vi "Init Commands.vi"(8 "error in (no error)":errorcluster, 10 "Commands":refnum<class "Group Config.lvclass">, 11 "DAQmxAI in":refnum<class "DAQmxAI.lvclass">) -> (0 "error out":errorcluster, 3 "DAQmxAI out":refnum<class "DAQmxAI.lvclass">)   [LabVIEW 2023, in "VolatusDAQ.lvlib" / "DAQmxAI.lvclass"]
uses:
  DAQmxAI.lvclass
  C:/dev/volatus/mts-volatus-super/libs/lv-volatus/Volatus/Module/Module.lvclass
  VolatusConfig/Group/Group Config.lvclass
  lv-vecto/Vecto/Group DBL/Group DBL.lvclass
  C:/dev/volatus/mts-volatus-super/libs/lv-vecto/Vecto/Group/Group.lvclass
  Cmd Index.ctl
  VolatusConfig/VolatusConfigElement/VolatusConfigElement.lvclass/VolatusConfigElement.ctl
  DAQmxAI.lvclass/DAQmxAI.ctl
  VolatusConfig/VolatusConfigElement/Element.vi
  VolatusConfig/Channel/Channel Config.lvclass
  C:/dev/volatus/mts-volatus-super/libs/lv-volatus/VolatusConfig/VolatusConfigElement/VolatusConfigElement.lvclass
  VolatusConfig/VolatusConfigElement/VolatusConfigElement.lvclass
  Volatus/Module/Module.lvclass
  C:/dev/volatus/mts-volatus-super/libs/lv-volatus/VolatusConfig/Channel/Channel Config.lvclass
  C:/dev/volatus/mts-volatus-super/libs/lv-vecto/Vecto/Group DBL/Group DBL.lvclass
  C:/dev/volatus/mts-volatus-super/libs/lv-volatus/VolatusDAQ/DAQmxAI/DAQmxAI.lvclass
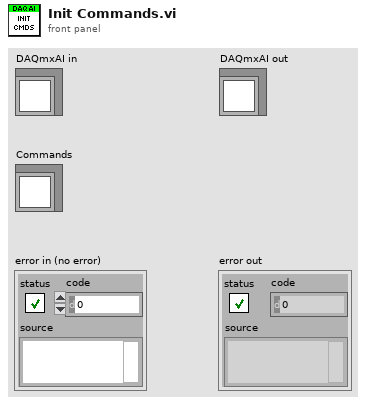
[diagram p1: front panel]
types:
  T1 = typedef "VolatusDAQ.lvlib/DAQmxAI.lvclass/Cmd Index.ctl" = cluster{"Null Offset":i32}
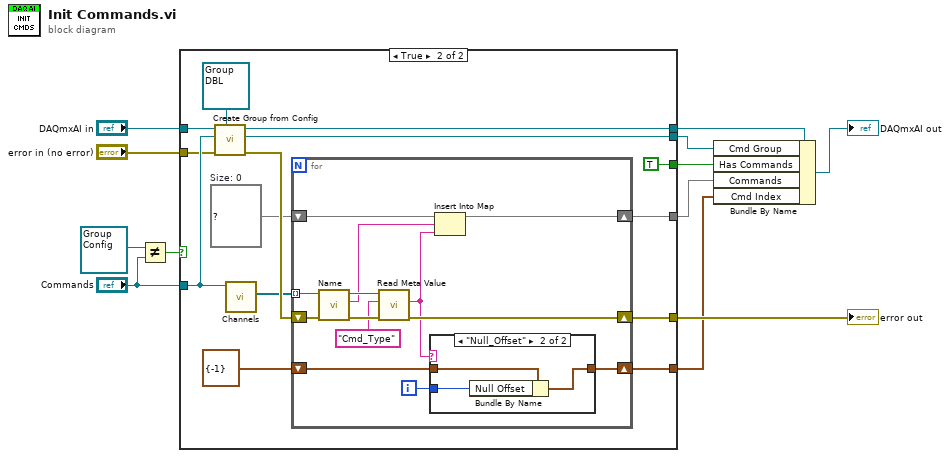
[diagram p0: block diagram]
diagram:
  n1 = Not Equal?(x=refnum<class "Group Config.lvclass"> refnum, y="Commands") -> (x != y?=w11:bool)
  n2 = case shown="True" w11 {
    tunnel: "Commands" -> [_ w22]
    tunnel: [_ w25] -> w2
    tunnel: "DAQmxAI in" -> [w14 w23]
    tunnel: [w13 w21] -> w4
    tunnel: [w14 w20] -> w8
    tunnel: [_ w19] -> w7
    tunnel: "error in (no error)" -> [w13 w18]
    tunnel: [_ w16] -> w3
    tunnel: [_ TRUE] -> w1
    frame False {
      # "No commandable channels configured"
    }
    frame True {
      w26 = map{string, string} {}  # Size: 0
      n3 = call "Create Group from Config.vi"("Group Type (Abstract)"=refnum<class "Group DBL.lvclass"> refnum ("Vecto.lvlib:Group.lvclass"), "error in (no error)"=w18, "Group Config"=w22, "Module in"=w23) -> ("error out"=w28:errorcluster, "Group"=w19:refnum<class "Group DBL.lvclass">, "Module out"=w20:refnum<class "DAQmxAI.lvclass">)  [unwired: 5 in]
      n4 = call "Channels.vi"("Group in"=w22) -> ("Channels"=w27:refnum<class "Channel Config.lvclass">[])  [unwired: 8 in, 2 out]
      n5 = for {
        tunnel: w27 -> [w40] mode=indexing
        shift-right: [w36] -> w25
        shift-left: w26 -> [w37]
        shift-right: [w33] -> w21
        shift-left: w28 -> [w34]
        shift-right: [w30] -> w16
        shift-left: T1 {"Null Offset"=-1} ("Cmd Index") -> [w31]
        i -> [w32]
        n6 = call "Name.vi"("error in (no error)"=w34, "VolatusConfigElement in"=w40) -> ("error out"=w41:errorcluster, "Name"=w35:string, "VolatusConfigElement out"=w38:refnum<class "Channel Config.lvclass">)  [unwired: 7 in]
        n7 = call "Read Meta Value.vi"("error in (no error)"=w41, "Meta Name"="Cmd_Type", "VolatusConfigElement in"=w38) -> ("error out"=w33:errorcluster, "Meta Value"=w29:string)  [unwired: 6 in, 1 out]
        n8 = case shown="\"Null_Offset\"" w29 {
          tunnel: w32 -> [_ w44]
          tunnel: w31 -> [w42 w45]
          tunnel: [w42 w43] -> w30
          frame Default {
          }
          frame "Null_Offset" {
            n9 = Bundle By Name(cluster=w45, "Null Offset"=w44) -> (w43:T1)
          }
        }
        n10 = Insert Into Map(map in=w37, key=w35, value=w29) -> (map out=w36:map{string, string})  [unwired: 2 out]
      }
    }
  }
  "error out" <- w4
  n11 = Bundle By Name(cluster=w8, "Cmd Group"=w7, "Has Commands"=w1, "Commands"=w2, "Cmd Index"=w3) -> (→"DAQmxAI out":refnum<class "DAQmxAI.lvclass">)
